vi "Motion Profile Right Drive Control.vi"(10 "runMotionProfile?":bool) -> ()   [LabVIEW 2019]
uses:
  <vilib>/Rock Robotics/WPI/ThirdParty/Phoenix-LabVIEW/Motor Controller/Controls/CTRE_Phoenix_MotorControl_MotionProfileControlMode.ctl
panel:
  out "Is Motion Profile Finished?":bool
  out "Btm Mot Prof Count":i32
  out "Top Mot Prof Count":i32
  out "Mot Prof Active Is Valid":bool
  out "Mot Prof Active Is Last":bool
  out "Mot Prof  Has Under Run":bool
  out "Mot Prof  Is Under Run":bool
  out "Mot Prof Active Position":dbl
  out "Mot Prof Active Velocity":dbl
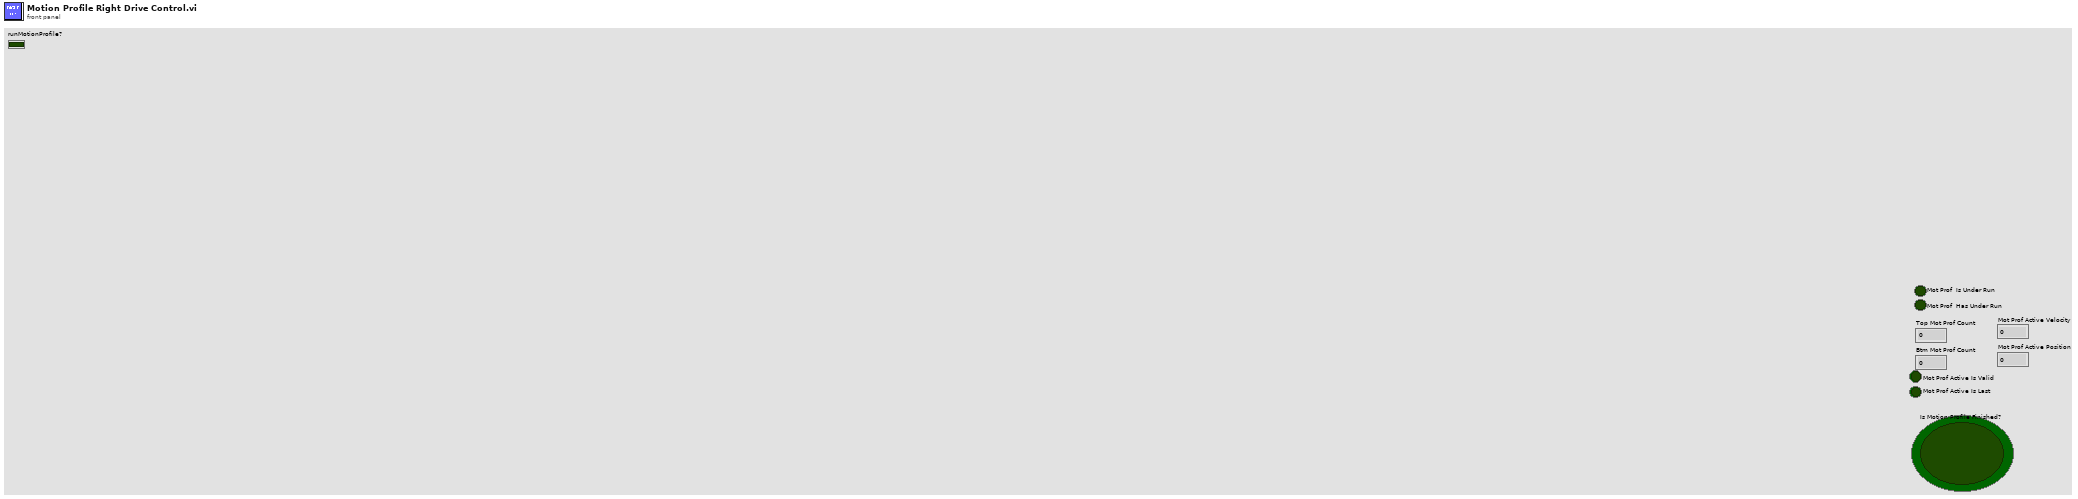
[diagram p1: front panel]
types:
  T1 = typedef "WPI_MotorControlDeviceRef.ctl" = cluster{"DeviceStatus":errorcluster, "Type":T2, "PWM":cluster{"PWM Channel":T3, "DeadBand":T4}, "CAN":cluster{"Device Number":u8, "SetOutput VI Ref":variant, "GetOutput VI Ref":variant, "Enable VI Ref":variant, "Disable VI Ref":variant, "Data":variant}, "Invert":bool, "DIO PWM":cluster{"PWM \"Enable\" Channel":T3, "DIOChannel":T5, "PWM Rate":dbl}}
  T2 = typedef "WPI_MotorControlType.ctl" = enum16{"PWM", "CAN", "DIO PWM"}
  T3 = typedef "FPGA_DIOPWMChannel.ctl" = enum8{"PWM 0", "PWM 1", "PWM 2", "PWM 3", "PWM 4", "PWM 5", "PWM 6", "PWM 7", "PWM 8", "PWM 9", "PWM MXP 0", "PWM MXP 1", "PWM MXP 2", "PWM MXP 3", "PWM MXP 4", "PWM MXP 5", "PWM MXP 6", "PWM MXP 7", "PWM MXP 8", "PWM MXP 9", "Invalid"}
  T4 = typedef "WPI_PWMDeadband.ctl" = cluster{"Name":string, "maxPositivePwm":i32, "minPositivePwm":i32, "centerPwm":i32, "maxNegativePwm":i32, "minNegativePwm":i32, "angularRange":u16}
  T5 = typedef "FPGA_DIOChannel.ctl" = enum8{"DIO 0", "DIO 1", "DIO 2", "DIO 3", "DIO 4", "DIO 5", "DIO 6", "DIO 7", "DIO 8", "DIO 9", "DIO MXP 0", "DIO MXP 1", "DIO MXP 2", "DIO MXP 3", "DIO MXP 4", "DIO MXP 5", "DIO MXP 6", "DIO MXP 7", "DIO MXP 8", "DIO MXP 9", "DIO MXP 10", "DIO MXP 11", "DIO MXP 12", "DIO MXP 13", "DIO MXP 14", "DIO MXP 15", "SPI Port CS1", "SPI Port CS2", "SPI Port CS3", "SPI Port MISO", "SPI Port MOSI", "Invalid"}
  T6 = cluster{"Top Buffer Remaining":i32, "Top Buffer Count":i32, "Bottom Buffer Count":i32, "Has Underrun?":bool, "Is Underrun?":bool, "Active Point Valid?":bool, "Is Last?":bool, "Profile Slot Select 0":i32, "Output Enable":i32, "Time Duration (ms)":i32, "Profile Slot Select 1":i32}
  T7 = typedef "CTRE_Phoenix_MotorControl_MotionProfileControlMode.ctl" = u16
  T8 = typedef "CTRE_Phoenix_MotorControl_BufferedTrajectoryPointStream_DeviceRef.ctl" = cluster{"Handle":u64, "Library Path":path}
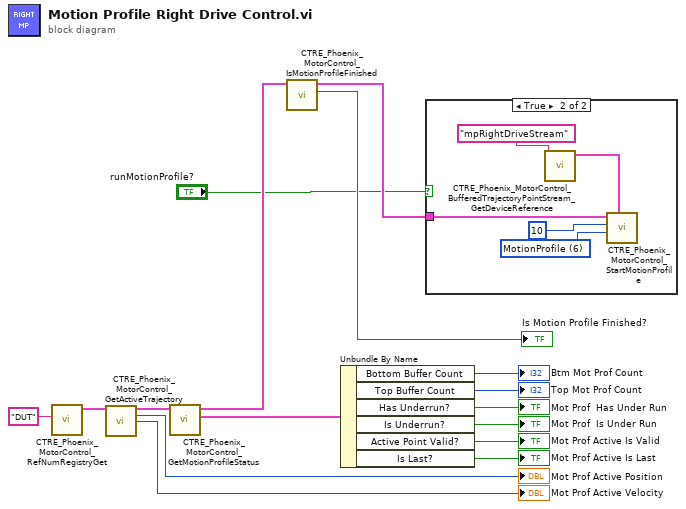
[diagram p0: block diagram]
diagram:
  n1 = call <vilib>:"CTRE_Phoenix_MotorControl_RefNumRegistryGet.vi"("refnum name"="DUT") -> ("PhoenixMotorControlDevRef"=w13:T1)  [unwired: 9 in, 1 out]
  n2 = call <vilib>:"CTRE_Phoenix_MotorControl_GetActiveTrajectory.vi"("PhoenixMotorControlDevRef"=w13) -> ("PhoenixMotorControlDevRef"=w5:T1, "Position (Sensor Units)"=→"Mot Prof Active Position":i32, "Velocity (Sensor Units per 100 ms)"=→"Mot Prof Active Velocity":i32)  [unwired: 10 in, 2 out]
  n3 = call <vilib>:"CTRE_Phoenix_MotorControl_GetMotionProfileStatus.vi"("PhoenixMotorControlDevRef"=w5) -> ("Motion Profile Status"=w12:T6, "PhoenixMotorControlDevRef"=w4:T1)  [unwired: 8 in, 1 out]
  n4 = call <vilib>:"CTRE_Phoenix_MotorControl_IsMotionProfileFinished.vi"("PhoenixMotorControlDevRef"=w4) -> ("Is Motion Profile Finished?"=→"Is Motion Profile Finished?":bool, "PhoenixMotorControlDevRef"=w2:T1)  [unwired: 8 in, 1 out]
  n5 = Unbundle By Name(w12) -> ("Bottom Buffer Count"=→"Btm Mot Prof Count":i32, "Top Buffer Count"=→"Top Mot Prof Count":i32, "Has Underrun?"=→"Mot Prof  Has Under Run":bool, "Is Underrun?"=→"Mot Prof  Is Under Run":bool, "Active Point Valid?"=→"Mot Prof Active Is Valid":bool, "Is Last?"=→"Mot Prof Active Is Last":bool)
  n6 = case shown="True" "runMotionProfile?" {
    tunnel: w2 -> [_ w17]
    frame False {
    }
    frame True {
      w21 = T7 6 items=["MotionProfile"=6, "MotionProfileArc"=10] ("Control Mode")
      n7 = call <vilib>:"CTRE_Phoenix_MotorControl_BufferedTrajectoryPointStream_GetDeviceReference.vi"("refnum name"="mpRightDriveStream") -> ("BufferedTrajectoryPointStream_DevRef"=w18:T8)  [unwired: 9 in, 1 out]
      n8 = call <vilib>:"CTRE_Phoenix_MotorControl_StartMotionProfile.vi"("BufferedTrajectoryPointStream_DevRef"=w18, "Control Mode"=w21, "minBufferedPts"=u32 10, "PhoenixMotorControlDevRef"=w17) -> ()  [unwired: 6 in, 2 out]
    }
  }
